vi "Create.vi"(10 "Channel":refnum<class "Channel.lvclass">) -> (3 "ChannelValue out":refnum<class "ChannelValue.lvclass">)   [LabVIEW 2020, in "Vecto.lvlib" / "ChannelValue.lvclass"]
uses:
  ChannelValue.lvclass
  Channel/Channel.lvclass
  ChannelValue.lvclass/ChannelValue.ctl
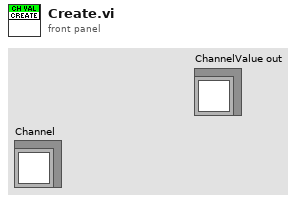
[diagram p1: front panel]
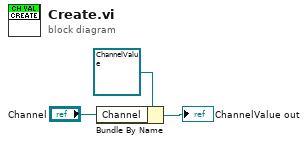
[diagram p0: block diagram]
diagram:
  n1 = Bundle By Name(cluster=refnum<class "ChannelValue.lvclass"> refnum ("ChannelValue in"), "Channel"="Channel") -> (→"ChannelValue out":refnum<class "ChannelValue.lvclass">)
